vi "MT Generate Fading profile.vi"   [LabVIEW 2020, in "niDMT.lvlib"]
doc: "Generates a user-specified Rayleigh or Rician fading profile for the complex baseband waveform. Call the MT Apply Fading Profile VI to apply the generated profile to a baseband I/Q waveform. You can use this VI for modeling Rayleigh and Rician fading profile distributions using Gans and Jakes models for characterizing flat-fading channels and time-varying frequency selective-fading channels."
uses:
  <vilib>/addons/Modulation/niDMT.lvlib
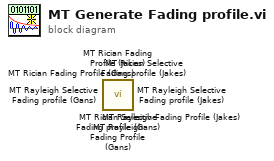
[diagram p0: block diagram]
diagram:
  n1 = call <vilib>:"MT Rician Selective Fading profile (Gans).vi"() -> ()  [unwired: 13 in, 3 out]
  n2 = call <vilib>:"MT Rician Selective Fading profile (Jakes).vi"() -> ()  [unwired: 13 in, 3 out]
  n3 = call <vilib>:"MT Rayleigh Selective Fading profile (Gans).vi"() -> ()  [unwired: 13 in, 3 out]
  n4 = call <vilib>:"MT Rayleigh Selective Fading profile (Jakes).vi"() -> ()  [unwired: 13 in, 3 out]
  n5 = call <vilib>:"MT Rician Fading Profile (Gans).vi"() -> ()  [unwired: 13 in, 3 out]
  n6 = call <vilib>:"MT Rician Fading Profile (Jakes).vi"() -> ()  [unwired: 13 in, 3 out]
  n7 = call <vilib>:"MT Rayleigh Fading Profile (Gans).vi"() -> ()  [unwired: 13 in, 3 out]
  n8 = call <vilib>:"MT Rayleigh Fading Profile (Jakes).vi"() -> ()  [unwired: 13 in, 3 out]
